vi "Task Information.vi"(11 "Refnum in":refnum<k21>) -> (3 "Array":T1(array[cluster]))   [LabVIEW 2017]
uses:
  <resource>/objmgr/daqmx.rc
panel:
  in  "error in (no error)":errorcluster
  out "error out":errorcluster
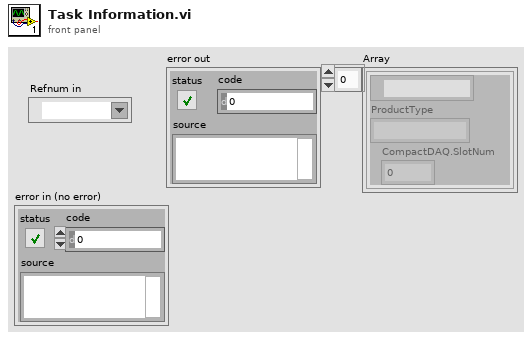
[diagram p1: front panel]
types:
  T1 = cluster{refnum<k21>, "ProductType":string, "CompactDAQ.SlotNum":u32}[]
  T2 = cluster{refnum<k21>, "ProductType":string, "CompactDAQ.SlotNum":u32}
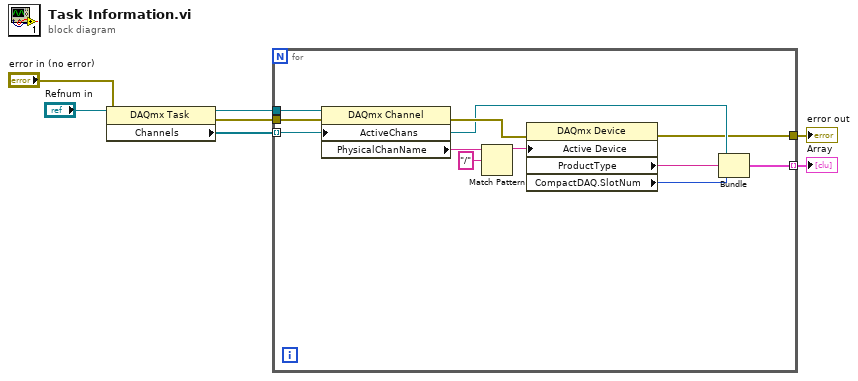
[diagram p0: block diagram]
diagram:
  n1 = property class="DAQmx Task"(reference="Refnum in", error in="error in (no error)") -> (reference out=w6:refnum<k21>, error out=w4:errorcluster, "Channels"=w5:refnum<k21>[])
  n2 = for {
    tunnel: w6 -> [w18]
    tunnel: w5 -> [w12] mode=indexing
    tunnel: w4 -> [w14]
    tunnel: [w9] -> w3 mode=indexing
    tunnel: [w8] -> w2
    n3 = property class="DAQmx Channel"(reference=w18, error in=w14, "ActiveChans"=w12) -> (error out=w13:errorcluster, "PhysicalChanName"=w17:tag)  [unwired: 1 out]
    n4 = Match Pattern(string=w17, regular expression="/") -> (before substring=w15:string)  [unwired: 1 in, 3 out]
    n5 = property class="DAQmx Device"(error in=w13, "Active Device"=w15) -> (error out=w8:errorcluster, "ProductType"=w11:string, "CompactDAQ.SlotNum"=w10:u32)  [unwired: 1 in, 1 out]
    n6 = Bundle(w12, "ProductType"=w11, "CompactDAQ.SlotNum"=w10) -> (w9:T2)  [unwired: 1 in]
  }
  "Array" <- w3
  "error out" <- w2
